vi "Nivel Global.vi"() -> ()   [LabVIEW 2014]
panel:
  in  "Nivel":bool
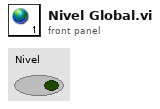
[diagram p1: front panel]
diagram:
